vi "Replace Doc by Index.vi"(0 "LV MDI in":refnum<class "LV MDI.lvclass">, 5 "Doc Class Object[]":refnum<class "Document.lvclass">[](array[class]), 7 "Doc index[]":i32[](array[numeric]), 11 "error in (no error)":errorcluster) -> (4 "LV MDI out":refnum<class "LV MDI.lvclass">, 15 "error out":errorcluster)   [LabVIEW 2016, in "LV MDI.lvclass"]
uses:
  LV MDI.lvclass
  Document/Document base/Document.lvclass
  LV MDI.lvclass/LV MDI.ctl
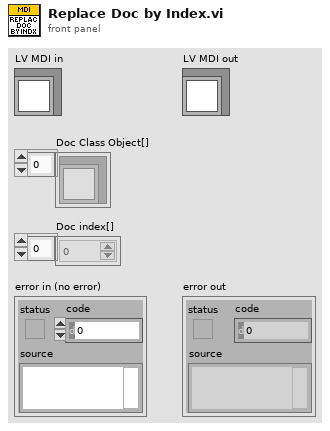
[diagram p1: front panel]
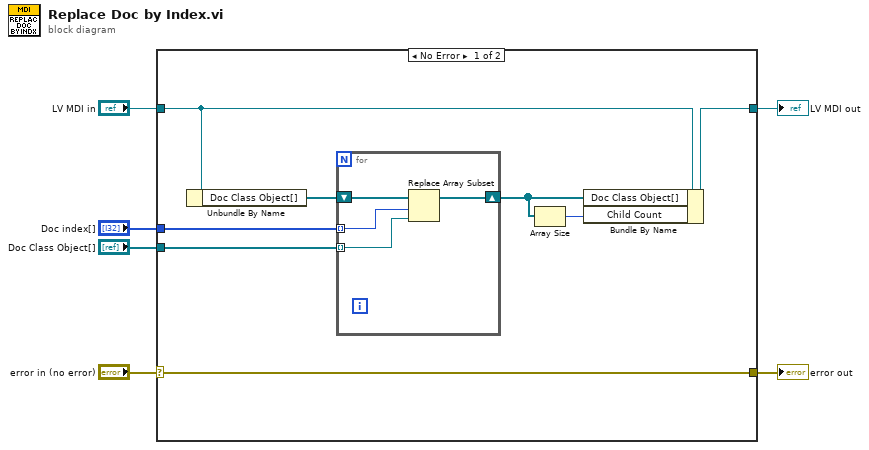
[diagram p0: block diagram]
diagram:
  n1 = case shown="No Error" "error in (no error)" {
    selector: "error in (no error)" -> [w14 w20]
    tunnel: [w14 w20] -> w5
    tunnel: [w10 w19] -> w3
    tunnel: "LV MDI in" -> [w11 w19]
    tunnel: "Doc index[]" -> [w13 _]
    tunnel: "Doc Class Object[]" -> [w7 _]
    frame No Error {
      n2 = Unbundle By Name(w11) -> ("Doc Class Object[]"=w12:refnum<class "Document.lvclass">[])
      n3 = for {
        tunnel: w13 -> [w16] mode=indexing
        tunnel: w7 -> [w15] mode=indexing
        shift-right: [w17] -> w8
        shift-left: w12 -> [w18]
        n4 = Replace Array Subset(array=w18, new element=w15, index=w16) -> (w17:refnum<class "Document.lvclass">[])
      }
      n5 = Array Size(array=w8) -> (size(s)=w9:i32)
      n6 = Bundle By Name(cluster=w11, "Doc Class Object[]"=w8, "Child Count"=w9) -> (w10:refnum<class "LV MDI.lvclass">)
    }
    frame Error {
    }
  }
  "error out" <- w5
  "LV MDI out" <- w3
